vi "Set Multiple Object Items.vi"(5 "Item Names":string[](array[string]), 6 "$Path or Item Name":string caption="Object $Path or Item Name", 7 "error in (no error)":errorcluster, 8 "JSON Items":string[](array[string]), 9 "Object Offset":i32, 10 "JSON":string="{}") -> (0 "error out":errorcluster, 3 "<JSON>":string)   [LabVIEW 2021, in "jsontext.facade.lvlib"]
doc: "Insert (or replace) multiple items into a JSON Object specified by the Object $Path. \n\nIf the path specified does not exist, but its immediate parent does, then a new object is created."
uses:
  jsontext.facade.lvlib
  jsontext/JSONtext.lvlib
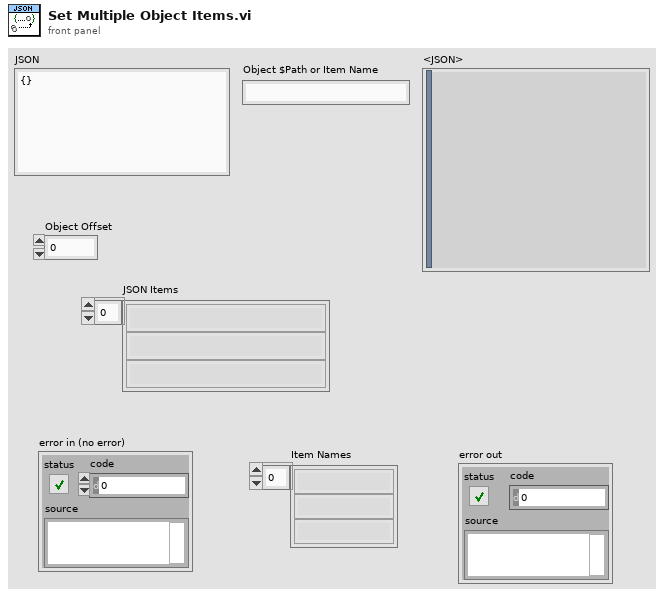
[diagram p1: front panel]
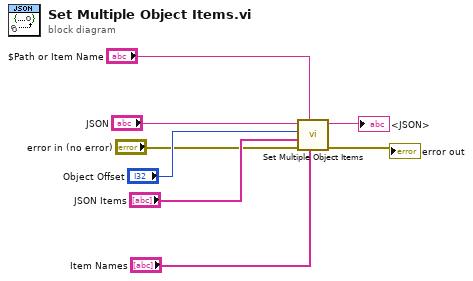
[diagram p0: block diagram]
diagram:
  n1 = call "Set Multiple Object Items.vi"("Item Names"="Item Names", "$Path or Item Name"="$Path or Item Name", "error in (no error)"="error in (no error)", "JSON Items"="JSON Items", "Object Offset"="Object Offset", "JSON"="JSON") -> ("error out"=→"error out":errorcluster, "<JSON>"=→"<JSON>":string)  [unwired: 3 in]
